vi "Disconnect.vi"(8 "error in (no error)":errorcluster, 11 "Sift Client in":refnum<class "Sift Client.lvclass">) -> (0 "error out":errorcluster, 3 "Sift Client out":refnum<class "Sift Client.lvclass">)   [LabVIEW 2024, in "Sift Client.lvlib" / "Sift Client.lvclass"]
doc: "Disconnect from Sift Proxy."
uses:
  Sift Client.lvclass
  Sift Client.lvclass/Sift Client.ctl
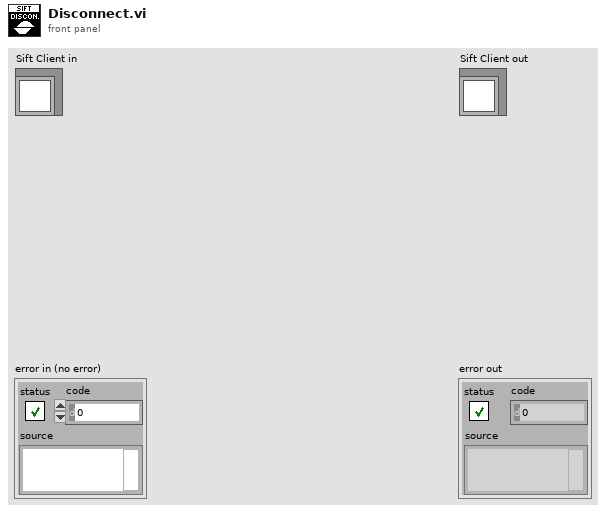
[diagram p1: front panel]
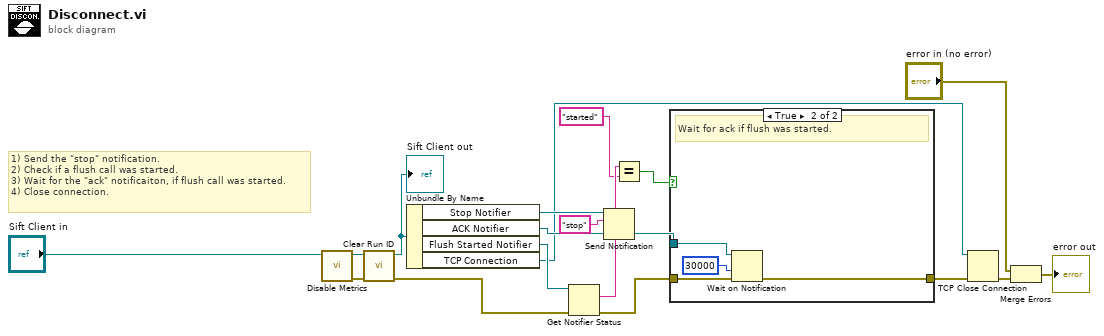
[diagram p0: block diagram]
diagram:
  # "1) Send the \"stop\" notification.\n2) Check if a flush call was started.\n3) Wait for the \"ack\" notificaiton, if flush call was started.\n4) Close connection."
  n1 = call-dynamic "Disable Metrics.vi"("Sift Client in"="Sift Client in") -> ("error out"=w2:errorcluster, "Sift Client out"=w5:refnum<class "Sift Client.lvclass">)  [unwired: 9 in]
  n2 = call-dynamic "Clear Run ID.vi"("error in (no error)"=w2, "Sift Client in"=w5) -> ("error out"=w1:errorcluster, "Sift Client out"=w3:refnum<class "Sift Client.lvclass">)  [unwired: 8 in]
  "Sift Client out" <- w3
  n3 = Unbundle By Name(w3) -> ("Stop Notifier"=w18:refnum<notifier>, "ACK Notifier"=w16:refnum<notifier>, "Flush Started Notifier"=w15:refnum<notifier>, "TCP Connection"=w10:refnum<k5>)
  n4 = Get Notifier Status(notifier=w15, error in (no error)=w1) -> (current notification=w14:string, error out=w11:errorcluster)  [unwired: 3 out]
  n5 = Send Notification(notification="stop", notifier=w18) -> ()  [unwired: 1 in, 2 out]
  n6 = Equal?(x=w14, y="started") -> (x = y?=w12:bool)
  n7 = case shown="True" w12 {
    tunnel: w16 -> [_ w23]
    tunnel: w11 -> [w19 w22]
    tunnel: [w19 w21] -> w6
    frame False {
      # "Flush wasn't started, skip waiting for ack."
    }
    frame True {
      # "Wait for ack if flush was started."
      n8 = Wait on Notification(notifier=w23, timeout in ms (-1)=30000, error in (no error)=w22) -> (error out=w21:errorcluster)  [unwired: 1 in, 3 out]
    }
  }
  n9 = TCP Close Connection(connection ID=w10, error in (no error)=w6) -> (error out=w9:errorcluster)  [unwired: 1 in, 1 out]
  n10 = Merge Errors("error in (no error)", w9) -> (→"error out":errorcluster)
